vi "chroma_serial_settings_to_labview_serial_settings.vi"(10 "CHR Serial settings":T1={"Baud rate"=enum."9600", "Parity"=enum."None", "Flow Ctrl"=enum."None"}) -> (2 "LV Serial settings":T2)   [LabVIEW 2015]
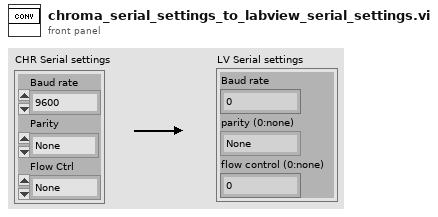
[diagram p1: front panel]
types:
  T1 = cluster{"Baud rate":enum32{"300", "600", "1200", "2400", "4800", "9600", "19200"}, "Parity":enum16{"None", "Odd", "Even"}, "Flow Ctrl":enum16{"None", "Software"}}
  T2 = cluster{"Baud rate":u32, "parity (0:none)":enum16{"None", "Odd", "Even", "Mark", "Space"}, "flow control (0:none)":u16}
  T3 = enum32{"300", "600", "1200", "2400", "4800", "9600", "19200"}
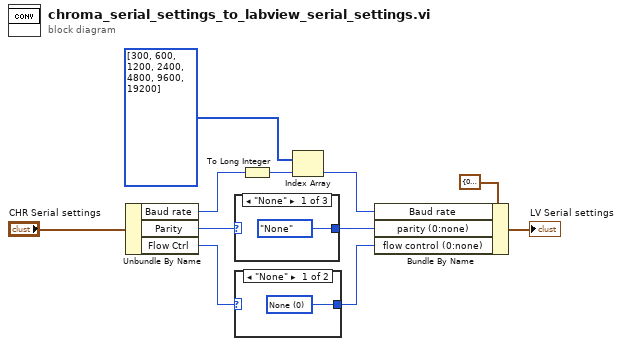
[diagram p0: block diagram]
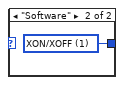
[diagram p2: hidden frame]
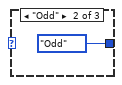
[diagram p3: hidden frame]
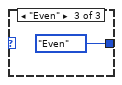
[diagram p4: hidden frame]
diagram:
  n1 = Unbundle By Name("CHR Serial settings") -> ("Baud rate"=w3:T3, "Parity"=w11:enum16{"None", "Odd", "Even"}, "Flow Ctrl"=w10:enum16{"None", "Software"})
  n2 = case shown="\"None\"" w11 {
    tunnel: [enum16{"None", "Odd", "Even", "Mark", "Space"}."None" ("parity (0:none)") enum16{"None", "Odd", "Even", "Mark", "Space"}."Odd" ("parity (0:none)") enum16{"None", "Odd", "Even", "Mark", "Space"}."Even" ("parity (0:none)")] -> w7
    frame "None" {
    }
    frame "Odd" {
    }
    frame "Even" {
    }
  }
  n3 = case shown="\"None\"" w10 {
    tunnel: [w15 w16] -> w8
    frame "None" {
      w15 = u16 0 items=["None", "XON/XOFF", "RTS/CTS", "XON/XOFF & RTS/CTS", "DTR/DSR", "XON/XOFF & DTR/DSR"] ("flow control (0:none)")
    }
    frame "Software" {
      w16 = u16 1 items=["None", "XON/XOFF", "RTS/CTS", "XON/XOFF & RTS/CTS", "DTR/DSR", "XON/XOFF & DTR/DSR"] ("flow control (0:none)")
    }
  }
  n4 = To Long Integer(number=w3) -> (32bit integer=w2:i32)
  n5 = Index Array(array=u32[] [300, 600, 1200, 2400, 4800, 9600, 19200], index=w2) -> (element=w1:u32)
  n6 = Bundle By Name(cluster=T2 {"Baud rate"=0, "parity (0:none)"=enum."Odd", "flow control (0:none)"=1}, "Baud rate"=w1, "parity (0:none)"=w7, "flow control (0:none)"=w8) -> (→"LV Serial settings":T2)
